vi "Set Pane Origin.vi"(8 "error in (no error)":errorcluster, 11 "VI in":refnum<vi>) -> (0 "error out":errorcluster)   [LabVIEW 2013, in "Utilities 1.lvlib"]
uses:
  Utilities 1.lvlib
  <vilib>/Utility/miscctls.llb/LVPointTypeDef.ctl
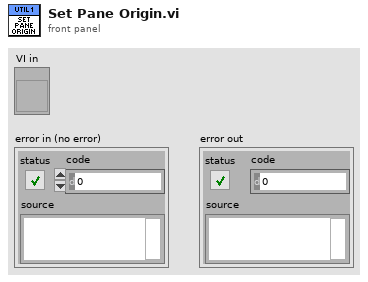
[diagram p1: front panel]
types:
  T1 = typedef "LVPointTypeDef.ctl" = cluster{"Horizontal":i16, "Vertical":i16}
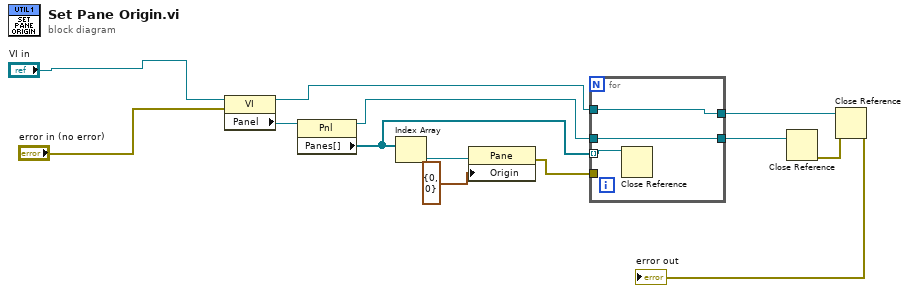
[diagram p0: block diagram]
diagram:
  n1 = property class="VI"(reference="VI in", error in="error in (no error)") -> (reference out=w9:refnum<vi>, "Panel"=w1:refnum<vi>)  [unwired: 1 out]
  n2 = property class="Pnl"(reference=w1) -> (reference out=w7:refnum<vi>, "Panes[]"=w4:refnum<vi>[])  [unwired: 1 in, 1 out]
  n3 = Index Array(array=w4) -> (element=w2:refnum<vi>)  [unwired: 1 in]
  n4 = property class="Pane"(reference=w2, "Origin"=T1 {"Horizontal"=0, "Vertical"=0}) -> (error out=w5:errorcluster)  [unwired: 1 in, 1 out]
  n5 = for {
    tunnel: w4 -> [w16] mode=indexing
    tunnel: w5 -> [_]
    tunnel: [w15] -> w6
    tunnel: w7 -> [w15]
    tunnel: [w14] -> w8
    tunnel: w9 -> [w14]
    n6 = Close Reference(reference=w16) -> ()  [unwired: 1 in, 1 out]
  }
  n7 = Close Reference(reference=w6) -> (error out=w10:errorcluster)  [unwired: 1 in]
  n8 = Close Reference(reference=w8, error in (no error)=w10) -> (error out=→"error out":errorcluster)
